vi "ManualSetParam.vi"(6 "Is":dbl, 7 "Int Time":i32, 8 "error in (no error)":errorcluster, 11 "Instruments in":refnum<class "Instruments.lvclass">) -> (0 "error out":errorcluster, 3 "Instruments out":refnum<class "Instruments.lvclass">)   [LabVIEW 2012, in "Instruments.lvclass"]
uses:
  Instruments.lvclass
  Instruments.lvclass/Instruments.ctl
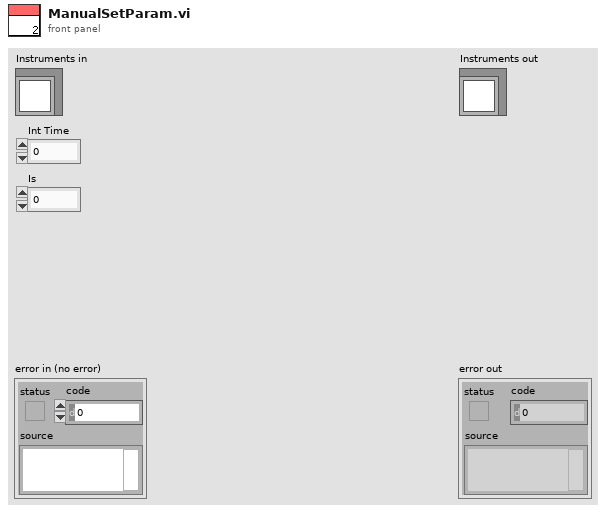
[diagram p1: front panel]
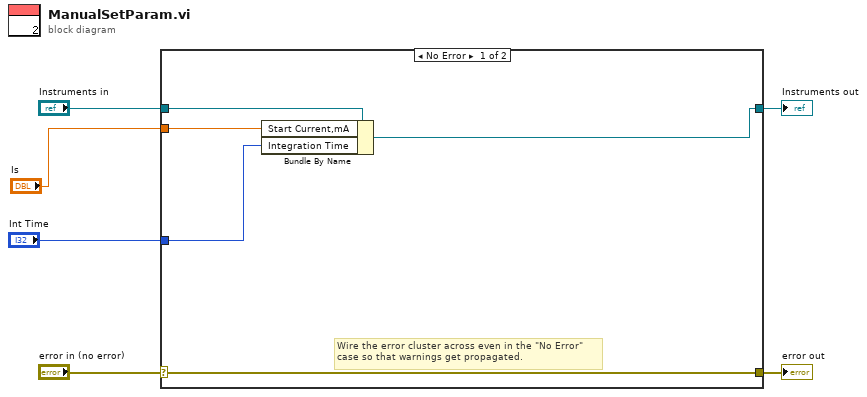
[diagram p0: block diagram]
diagram:
  n1 = case shown="No Error" "error in (no error)" {
    selector: "error in (no error)" -> [w11 w13]
    tunnel: [w11 w13] -> w5
    tunnel: [w8 w12] -> w3
    tunnel: "Instruments in" -> [w10 w12]
    tunnel: "Is" -> [w9 _]
    tunnel: "Int Time" -> [w7 _]
    frame No Error {
      # "Wire the error cluster across even in the \"No Error\"\ncase so that warnings get propagated."
      n2 = Bundle By Name(cluster=w10, "Start Current,mA"=w9, "Integration Time"=w7) -> (w8:refnum<class "Instruments.lvclass">)
    }
    frame Error {
    }
  }
  "error out" <- w5
  "Instruments out" <- w3
